vi "Advection_Sub.vi"(1 "Uref":dbl, 2 "Z":dbl) -> (0 "U m/s":dbl)   [LabVIEW 2010]
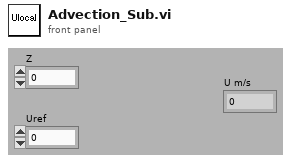
[diagram p1: front panel]
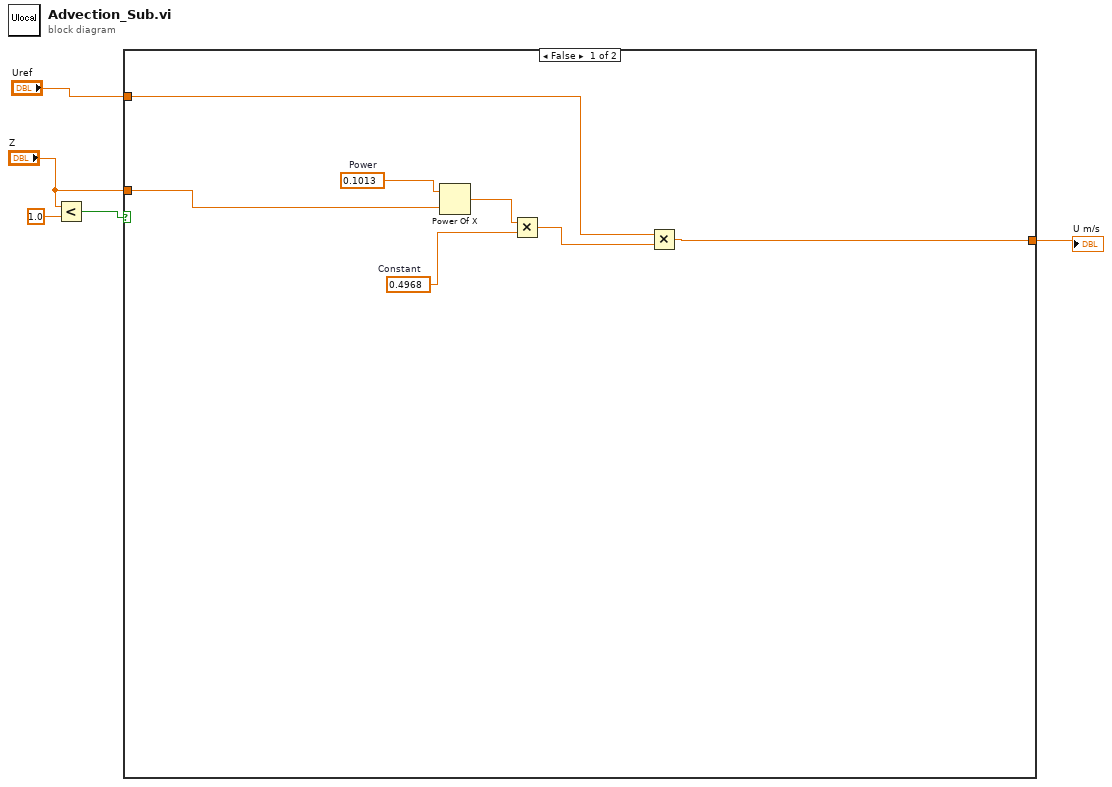
[diagram p0: block diagram]
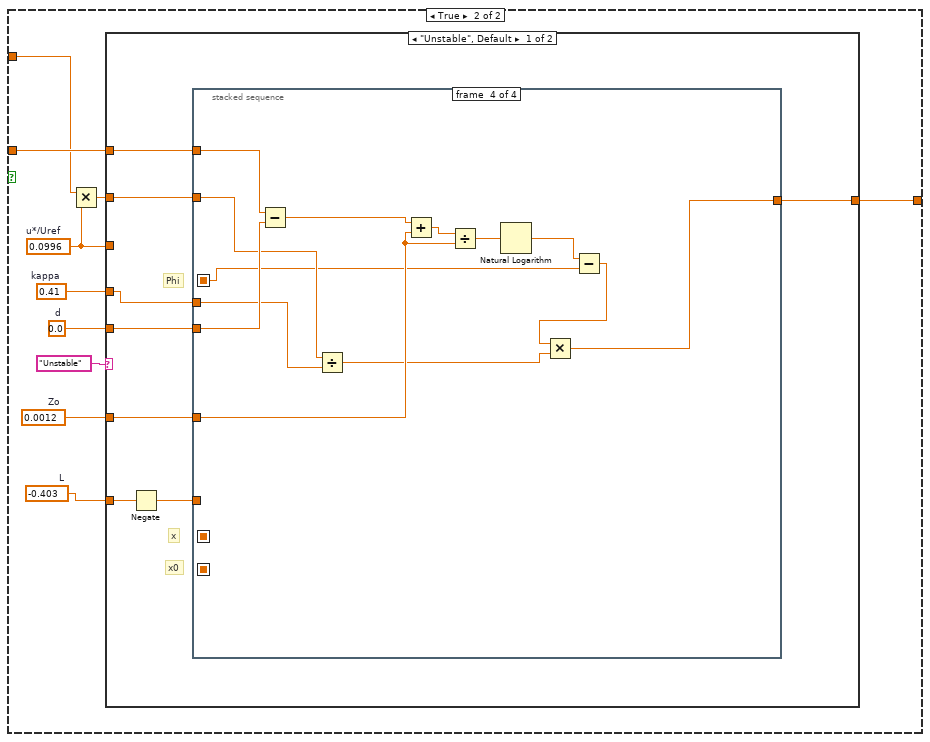
[diagram p2: hidden frame]
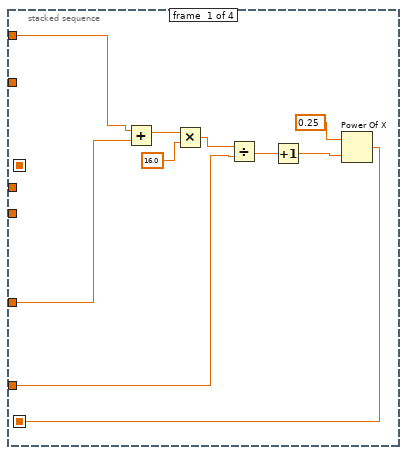
[diagram p3: hidden frame]
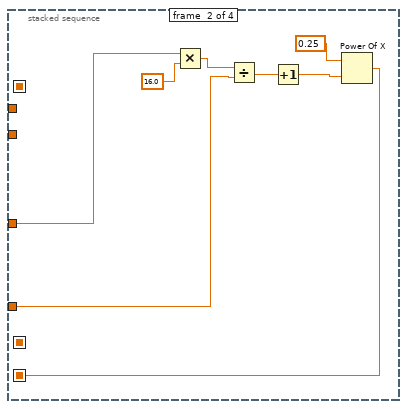
[diagram p4: hidden frame]
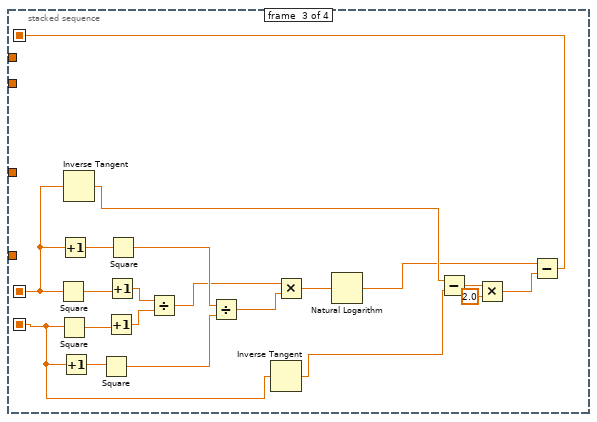
[diagram p5: hidden frame]
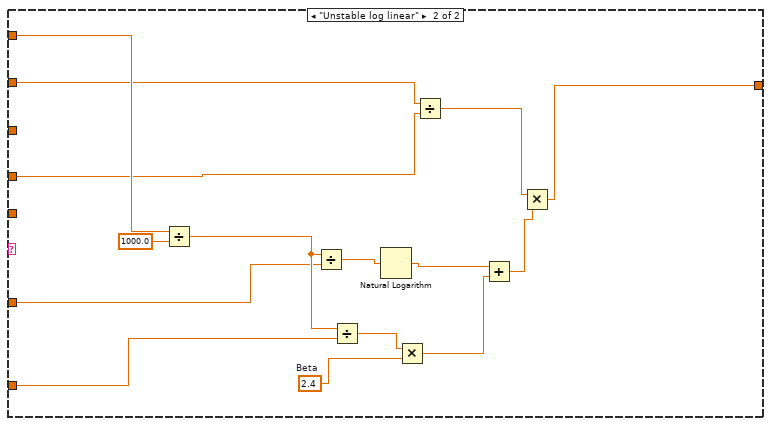
[diagram p6: hidden frame]
diagram:
  n1 = Less?(x="Z", y=1.0) -> (x < y?=w4:bool)
  n2 = case shown="False" w4 {
    tunnel: "Z" -> [w11 w21]
    tunnel: [w6 w22] -> w2
    tunnel: "Uref" -> [w7 w18]
    frame False {
      w9 = 0.4968  # Constant
      w12 = 0.1013  # Power
      n3 = Power Of X(1:w11, 2:w12) -> (0:w10:dbl)
      n4 = Multiply(x=w10, y=w9) -> (x*y=w8:dbl)
      n5 = Multiply(x=w7, y=w8) -> (x*y=w6:dbl)
    }
    frame True {
      w13 = 0.0  # d
      w14 = -0.403  # L
      w15 = 0.0012  # Zo
      w16 = 0.41  # kappa
      w19 = 0.0996  # u*/Uref
      n6 = Multiply(x=w18, y=w19) -> (x*y=w17:dbl)
      n7 = case shown="\"Unstable\", Default" "Unstable" {
        tunnel: [w23 w89] -> w22
        tunnel: w21 -> [w30 w88]
        tunnel: w19 -> [_ _]
        tunnel: w17 -> [w25 w85]
        tunnel: w16 -> [w24 w84]
        tunnel: w15 -> [w29 w83]
        tunnel: w14 -> [w28 w82]
        tunnel: w13 -> [w26 _]
        frame "Unstable", Default {
          # "Phi"
          # "x0"
          # "x"
          n8 = Negate(x=w28) -> (-x=w27:dbl)
          n9 = stacked-sequence {
            seq-local: [w31 _ _ _] -> [_ _ w57 _]
            seq-local: [_ w41 _ _] -> [_ _ w56 _]
            seq-local: [_ _ w49 _] -> [_ _ _ w71]
            tunnel: w30 -> [w40 _ _ w81]
            tunnel: w29 -> [w39 w42 _ w75]
            tunnel: w27 -> [w35 w46 _ _]
            tunnel: w26 -> [_ _ _ w80]
            tunnel: w25 -> [_ _ _ w79]
            tunnel: w24 -> [_ _ _ w78]
            tunnel: [_ _ _ w69] -> w23
            frame #0 {
              n10 = Add(x=w40, y=w39) -> (x+y=w38:dbl)
              n11 = Multiply(x=w38, y=16.0) -> (x*y=w36:dbl)
              n12 = Divide(x=w36, y=w35) -> (x/y=w34:dbl)
              n13 = Increment(x=w34) -> (x+1=w33:dbl)
              n14 = Power Of X(1:w33, 2:0.25 ("y")) -> (0:w31:dbl)
            }
            frame #1 {
              n15 = Multiply(x=w42, y=16.0) -> (x*y=w47:dbl)
              n16 = Divide(x=w47, y=w46) -> (x/y=w45:dbl)
              n17 = Increment(x=w45) -> (x+1=w44:dbl)
              n18 = Power Of X(1:w44, 2:0.25 ("y")) -> (0:w41:dbl)
            }
            frame #2 {
              n19 = Square(x=w57) -> (x^2=w66:dbl)
              n20 = Square(x=w56) -> (x^2=w65:dbl)
              n21 = Increment(x=w57) -> (x+1=w68:dbl)
              n22 = Increment(x=w56) -> (x+1=w67:dbl)
              n23 = Inverse Tangent(1:w57) -> (0:w55:dbl)
              n24 = Square(x=w67) -> (x^2=w63:dbl)
              n25 = Increment(x=w65) -> (x+1=w61:dbl)
              n26 = Increment(x=w66) -> (x+1=w62:dbl)
              n27 = Square(x=w68) -> (x^2=w64:dbl)
              n28 = Divide(x=w62, y=w61) -> (x/y=w59:dbl)
              n29 = Divide(x=w64, y=w63) -> (x/y=w60:dbl)
              n30 = Inverse Tangent(1:w56) -> (0:w54:dbl)
              n31 = Multiply(x=w59, y=w60) -> (x*y=w58:dbl)
              n32 = Natural Logarithm(1:w58) -> (0:w50:dbl)
              n33 = Subtract(x=w55, y=w54) -> (x-y=w53:dbl)
              n34 = Multiply(x=w53, y=2.0) -> (x*y=w51:dbl)
              n35 = Subtract(x=w50, y=w51) -> (x-y=w49:dbl)
            }
            frame #3 {
              n36 = Subtract(x=w81, y=w80) -> (x-y=w77:dbl)
              n37 = Divide(x=w79, y=w78) -> (x/y=w73:dbl)
              n38 = Add(x=w77, y=w75) -> (x+y=w76:dbl)
              n39 = Divide(x=w76, y=w75) -> (x/y=w74:dbl)
              n40 = Natural Logarithm(1:w74) -> (0:w72:dbl)
              n41 = Subtract(x=w72, y=w71) -> (x-y=w70:dbl)
              n42 = Multiply(x=w70, y=w73) -> (x*y=w69:dbl)
            }
          }
        }
        frame "Unstable log linear" {
          w94 = 2.4  # Beta
          n43 = Divide(x=w88, y=1000.0) -> (x/y=w87:dbl)
          n44 = Divide(x=w87, y=w83) -> (x/y=w96:dbl)
          n45 = Divide(x=w87, y=w82) -> (x/y=w93:dbl)
          n46 = Natural Logarithm(1:w96) -> (0:w95:dbl)
          n47 = Multiply(x=w93, y=w94) -> (x*y=w92:dbl)
          n48 = Divide(x=w85, y=w84) -> (x/y=w90:dbl)
          n49 = Add(x=w95, y=w92) -> (x+y=w91:dbl)
          n50 = Multiply(x=w90, y=w91) -> (x*y=w89:dbl)
        }
      }
    }
  }
  "U m/s" <- w2
